vi "write_temperature(SubVI).vi"(8 "error in (no error)":errorcluster, 10 "read buffer":string, 11 "VISA Refnum in":refnum<visa-resource-name>) -> (0 "error out":errorcluster, 3 "VISA Refnum out":refnum<visa-resource-name>)   [LabVIEW 2018]
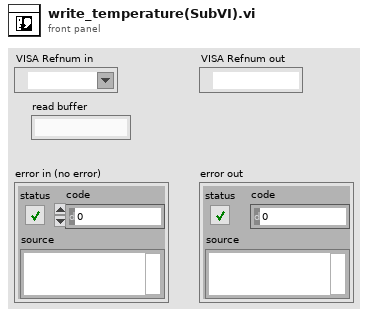
[diagram p1: front panel]
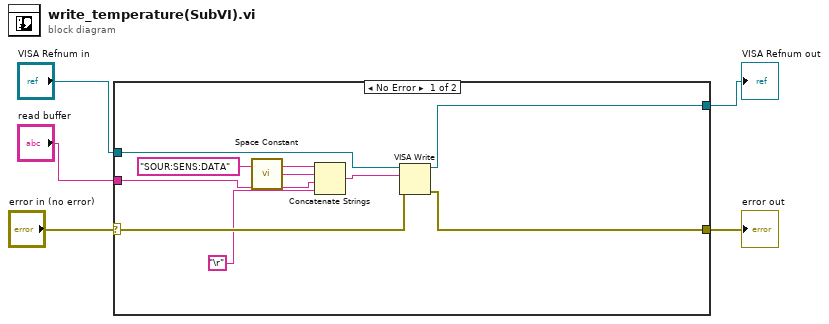
[diagram p0: block diagram]
diagram:
  n1 = case shown="No Error" "error in (no error)" {
    selector: "error in (no error)" -> [w9 w15]
    tunnel: [w14 w15] -> w5
    tunnel: [w13 _] -> w4
    tunnel: "VISA Refnum in" -> [w10 _]
    tunnel: "read buffer" -> [w6 _]
    frame No Error {
      n2 = call <vilib>:"Space Constant.vi"() -> ("String"=w7:string)
      n3 = Concatenate Strings("SOUR:SENS:DATA" ("string"), w7, w6, "\r") -> (w12:string)
      n4 = VISA Write(VISA resource name=w10, write buffer=w12, error in (no error)=w9) -> (VISA resource name out=w13:refnum<visa-resource-name>, error out=w14:errorcluster)  [unwired: 1 out]
    }
    frame Error {
    }
  }
  "error out" <- w5
  "VISA Refnum out" <- w4
